vi "Calculate Cubic Bezier.vi"(7 "Iterations":i32=10000, 9 "error in (no error)":errorcluster, 11 "Points":T1[](array[typedef])) -> (1 "error out":errorcluster, 2 "Y":dbl[](array[numeric]), 3 "X":dbl[](array[numeric]))   [LabVIEW 2019, in "Tool Path.lvclass"]
uses:
  Tool Path.lvclass
  Parse/PathCommands/Point.ctl
  Parse/PathCommands/PathCommands.lvclass
panel:
  out "Time":u32
  # "M 190,440\nC 250,385 310,330 415,350 350,390 270,420 250,540"
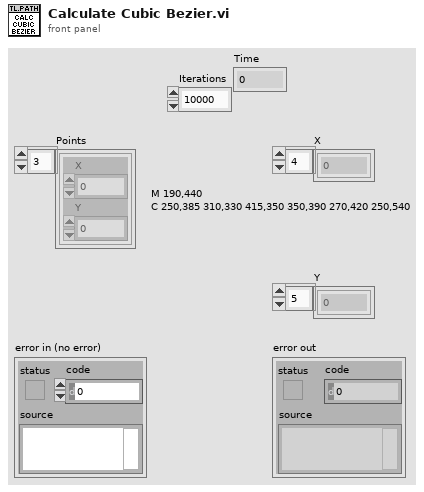
[diagram p1: front panel]
types:
  T1 = typedef "PathCommands.lvclass/Point.ctl" = cluster{"X":dbl, "Y":dbl}
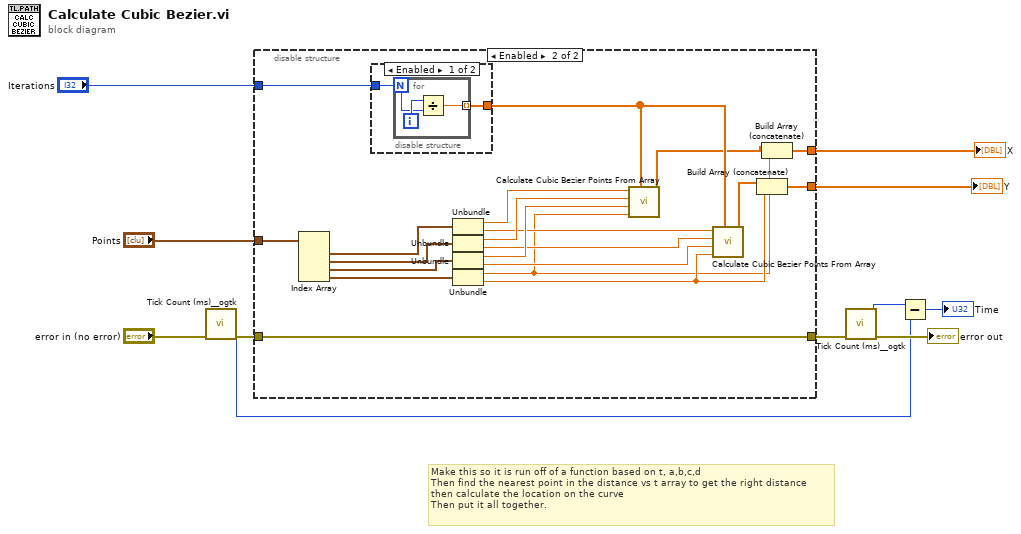
[diagram p0: block diagram]
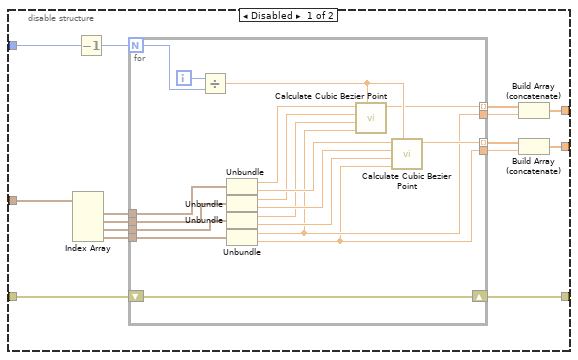
[diagram p2: hidden frame]
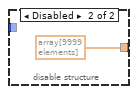
[diagram p3: hidden frame]
diagram:
  # "Make this so it is run off of a function based on t, a,b,c,d\nThen find the nearest point in the distance vs t array to get the right distance\nthen calculate the location on the curve\nThen put it all together."
  n1 = call <userlib>:"Tick Count (ms)__ogtk.vi"("error in (no error)"="error in (no error)") -> ("error out"=w5:errorcluster, "millisecond timer value"=w2:u32)  [unwired: 9 in]
  n2 = disable-structure shown="Enabled" {
    disable-tunnel: [w26 w59] -> w11
    disable-tunnel: w5 -> [w25 w59]
    disable-tunnel: "Iterations" -> [w20 w58]
    disable-tunnel: [w18 w50] -> w8
    disable-tunnel: [w14 w45] -> w7
    disable-tunnel: "Points" -> [w12 w60]
    frame Disabled {
      n3 = Index Array(array=w12) -> (element #1=w24:T1, element #2=w23:T1, element #3=w22:T1, element #4=w21:T1)  [unwired: 4 in]
      n4 = Decrement(x=w20) -> (x-1=w13:i32)
      n5 = for {
        N: w13 -> [w42]
        shift-right: [w44] -> w26
        shift-left: w25 -> [w44]
        tunnel: w24 -> [w31]
        tunnel: w23 -> [w30]
        tunnel: w22 -> [w29]
        tunnel: w21 -> [w40]
        tunnel: [w39] -> w15 mode=indexing
        tunnel: [w38] -> w19 mode=indexing
        tunnel: [w27] -> w17
        tunnel: [w28] -> w16
        i -> [w43]
        n6 = Divide(x=w43, y=w42) -> (x/y=w41:dbl)
        n7 = Unbundle(w31) -> ("X"=w32:dbl, "Y"=w35:dbl)
        n8 = Unbundle(w30) -> ("X"=w34:dbl, "Y"=w36:dbl)
        n9 = Unbundle(w29) -> ("X"=w33:dbl, "Y"=w37:dbl)
        n10 = Unbundle(w40) -> ("X"=w28:dbl, "Y"=w27:dbl)
        n11 = call "Calculate Cubic Bezier Point.vi"("t"=w41, "d"=w28, "c"=w33, "b"=w34, "a"=w32) -> ("f(t)"=w39:dbl)  [unwired: 6 in]
        n12 = call "Calculate Cubic Bezier Point.vi"("t"=w41, "d"=w27, "c"=w37, "b"=w36, "a"=w35) -> ("f(t)"=w38:dbl)  [unwired: 6 in]
      }
      n13 = Build Array (concatenate)(w15, w16) -> (w14:dbl[])
      n14 = Build Array (concatenate)(w19, w17) -> (w18:dbl[])
    }
    frame Enabled {
      n15 = Index Array(array=w60) -> (element #1=w61:T1, element #2=w62:T1, element #3=w63:T1, element #4=w64:T1)  [unwired: 4 in]
      n16 = disable-structure shown="Enabled" {
        disable-tunnel: w58 -> [w66 _]
        disable-tunnel: [w65 dbl[] array[9999 elements] ("Array")] -> w51
        frame Enabled {
          n17 = for {
            N: w66 -> [w68]
            tunnel: [w67] -> w65 mode=indexing
            i -> [w69]
            n18 = Divide(x=w69, y=w68) -> (x/y=w67:dbl)
          }
        }
        frame Disabled {
        }
      }
      n19 = Unbundle(w61) -> ("X"=w55:dbl, "Y"=w52:dbl)
      n20 = Unbundle(w62) -> ("X"=w57:dbl, "Y"=w53:dbl)
      n21 = Unbundle(w63) -> ("X"=w56:dbl, "Y"=w54:dbl)
      n22 = Unbundle(w64) -> ("X"=w47:dbl, "Y"=w49:dbl)
      n23 = call "Calculate Cubic Bezier Points From Array.vi"("t"=w51, "d"=w47, "c"=w56, "b"=w57, "a"=w55) -> ("f(t)"=w46:dbl[])  [unwired: 6 in]
      n24 = call "Calculate Cubic Bezier Points From Array.vi"("t"=w51, "d"=w49, "c"=w54, "b"=w53, "a"=w52) -> ("f(t)"=w48:dbl[])  [unwired: 6 in]
      n25 = Build Array (concatenate)(w48, w49) -> (w50:dbl[])
      n26 = Build Array (concatenate)(w46, w47) -> (w45:dbl[])
    }
  }
  "X" <- w7
  "Y" <- w8
  n27 = call <userlib>:"Tick Count (ms)__ogtk.vi"("error in (no error)"=w11) -> ("error out"=→"error out":errorcluster, "millisecond timer value"=w3:u32)  [unwired: 9 in]
  n28 = Subtract(x=w3, y=w2) -> (x-y=→"Time":u32)
